vi "CAN Stop Schedule.vi"(10 "CANIndex":u8, 11 "DevHandle":i32) -> (3 "function return":i32)   [LabVIEW 2010, in "usb2can.lvlib"]
doc: "int WINAPI CAN_StopSchedule(int DevHandle, unsigned char CANIndex);"
uses:
  usb2can.lvlib
  USB2XXX.dll
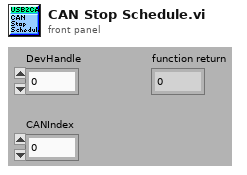
[diagram p1: front panel]
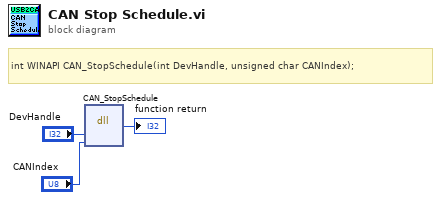
[diagram p0: block diagram]
diagram:
  # "int WINAPI CAN_StopSchedule(int DevHandle, unsigned char CANIndex);"
  n1 = dll-call lib="E:/Projects/USB2XXX_Example/sdk/api/Labview/usb2can/USB2XXX.*" fn="CAN_StopSchedule"("DevHandle"="DevHandle", "CANIndex"="CANIndex") -> (→"function return":i32)  [unwired: 5 in, 2 out]
